vi "No TitleBar FP.vi"() -> ()   [LabVIEW 2019]
panel:
  in  "Title":string="My Frameless App"
  in  "Stop":bool
  out "Waveform Graph":waveform(dbl)(graph)
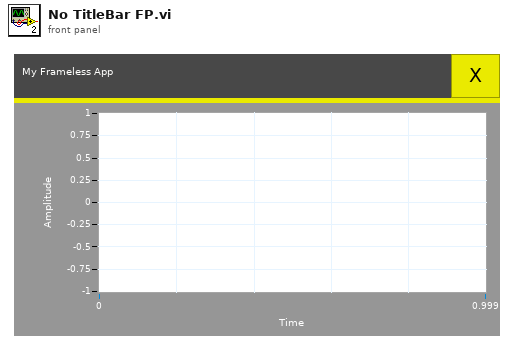
[diagram p1: front panel]
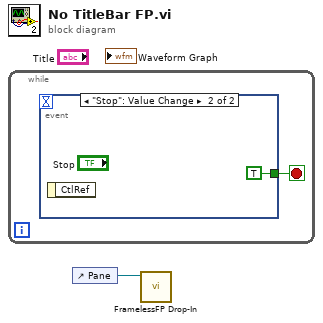
[diagram p0: block diagram]
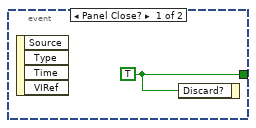
[diagram p2: hidden frame]
diagram:
  n1 = while {
    stop <- w2 stop-if-true
    n2 = event shown="[1] \"Stop\": Value Change" {
      selector: _ -> [_ _]
      dyn-events: _ -> [_ _]
      timeout: _ -> [_ _]
      tunnel: [w3 TRUE ("Discard?")] -> w2
      event Panel Close? {
        w3 = TRUE ("Discard?")
        n3 = event-data() -> ()  [unwired: 1 in, 4 out]
        n4 = event-data("Discard?"=w3) -> ()  [unwired: 1 in, 1 out]
      }
      event "Stop": Value Change {
        n5 = event-data() -> ()  [unwired: 1 in, 1 out]
      }
    }
  }
  n6 = control-ref of="Pane"() -> (w1:refnum<vi>)
  n7 = call "FramelessFP Drop-In.vi"("Pane in"=w1) -> ()  [unwired: 10 in, 1 out]
